vi "VI Tree.vi"   [LabVIEW 2013]
doc: "This is the instrument driver for the Agilent 34401/34410/34411 digital multimeter."
uses:
  TD Algorithm Information.ctl
  TD Uncertainty Calculation Method.ctl
  TD Correlation Calculation Settings.ctl
  TD DOF Calculation Settings.ctl
  TD MCM Calculation Method.ctl
  TD MCM Calculation Settings.ctl
  TD Calculation Settings.ctl
  TD Quantity.ctl
panel:
  # "SEE DIAGRAM\nFOR VI Tree"
types:
  T1 = typedef "TD Quantity.ctl" = cluster{"Name":string, "Value":dbl[][], "Uncertainty":dbl[][], "Degrees of\nFreedom":dbl[][], "Correlation":dbl[][], "Randomized uncertainty":dbl[][]}
  T2 = typedef "TD Calculation Settings.ctl" = cluster{"Verbose":bool, "Uncertainty Calculation Method":T3, "Correlations":T4, "Degrees of Freedom":T5, "MCM Calculation Settings":T6}
  T3 = typedef "TD Uncertainty Calculation Method.ctl" = enum16{"none", "GUF", "MCM"}
  T4 = typedef "TD Correlation Calculation Settings.ctl" = cluster{"Required":bool, "Generate":bool}
  T5 = typedef "TD DOF Calculation Settings.ctl" = cluster{"Required":bool, "Generate":bool}
  T6 = typedef "TD MCM Calculation Settings.ctl" = cluster{"Repeats":i32, "Verbose":bool, "Parallelization method":T7, "Processors":i32, "Temporary directory":string, "Randomize":bool}
  T7 = typedef "TD MCM Calculation Method.ctl" = enum16{"Single Core", "Multi Core", "Multi Station"}
  T8 = typedef "TD Algorithm Information.ctl" = cluster{"ID":string, "Name":string, "Description":string, "Citation":string, "Remarks":string, "License":string, "Requires":string[], "Requires - description":string[], "Returns":string[], "Returns - description":string[], "Provides GUF":bool, "Provides MCM":bool, "Full path":string}
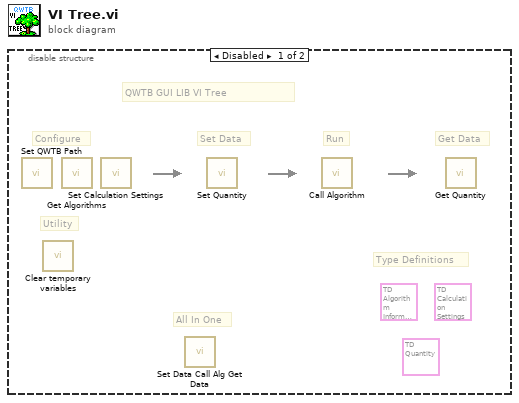
[diagram p0: block diagram]
diagram:
  n1 = disable-structure shown="Disabled" {
    frame Disabled {
      (unwired) T1 {"Name"="", "Value"=[[1.0]], "Uncertainty"=[[1.0]], "Degrees of\nFreedom"=[[10.0]], "Correlation"=[[10.0]], "Randomized uncertainty"=[[10.0]]} ("Quantity")
      (unwired) T2 {"Verbose"=TRUE, "Uncertainty Calculation Method"=enum."none", "Correlations"={"Required"=FALSE, "Generate"=TRUE}, "Degrees of Freedom"={"Required"=TRUE, "Generate"=TRUE}, "MCM Calculation Settings"={"Repeats"=100, "Verbose"=TRUE, "Parallelization method"=enum."Single Core", "Processors"=1, "Temporary directory"=".", "Randomize"=TRUE}} ("Calculation Settings")
      (unwired) T8 {"ID"="", "Name"="", "Description"="", "Citation"="", "Remarks"="", "License"="", "Requires"=[], "Requires - description"=[], "Returns"=[], "Returns - description"=[], "Provides GUF"=FALSE, "Provides MCM"=FALSE, "Full path"=""} ("Algorithm Information")
      # "QWTB GUI LIB VI Tree"
      # "Type Definitions"
      # "Set Data"
      # "All In One"
      # "Configure"
      # "Utility"
      # "Get Data"
      # "Run"
      n2 = call "Set QWTB Path.vi"() -> ()  [unwired: 11 in, 1 out]
      n3 = call "Clear temporary variables.vi"() -> ()  [unwired: 11 in, 1 out]
      n4 = call "Get Algorithms.vi"() -> ()  [unwired: 10 in, 2 out]
      n5 = call "Set Calculation Settings.vi"() -> ()  [unwired: 11 in, 1 out]
      n6 = call "Set Data Call Alg Get Data.vi"() -> ()  [unwired: 10 in, 2 out]
      n7 = call "Set Quantity.vi"() -> ()  [unwired: 11 in, 1 out]
      n8 = call "Call Algorithm.vi"() -> ()  [unwired: 11 in, 1 out]
      n9 = call "Get Quantity.vi"() -> ()  [unwired: 10 in, 2 out]
    }
    frame Enabled {
    }
  }
